vi "DO输出.vi"(8 "错误输入（无错误）":errorcluster, 9 "TF":bool=TRUE, 10 "序号":i32=19) -> (0 "错误输出":errorcluster)   [LabVIEW 2012]
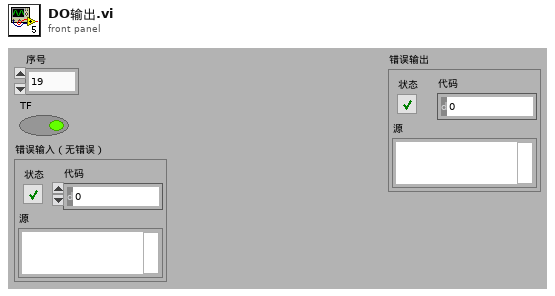
[diagram p1: front panel]
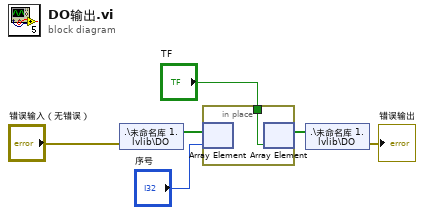
[diagram p0: block diagram]
diagram:
  n1 = shared-variable ".\\未命名库 1.lvlib\\DO"(error in="错误输入（无错误）") -> (w6:bool[])  [unwired: 1 out]
  n2 = in-place {
    in-place-border: "TF" -> [w7]
    n3 = in-place-array #1(w6, "序号") -> ()  [unwired: 1 out]
    n4 = in-place-array #1(w7) -> (w5:bool[])  [unwired: 1 out]
  }
  n5 = shared-variable ".\\未命名库 1.lvlib\\DO"(w5) -> (error out=→"错误输出":errorcluster)  [unwired: 1 in]
